vi "Read Discrete Inputs Request.vi"(8 "error in (no error)":errorcluster, 9 "number of inputs":u16, 10 "starting address":u16) -> (0 "error out":errorcluster, 1 "Modbus Data Unit out":T1={"function"=1, "Data"=[]} {"function" items=["Read Discrete Inputs"=2, "Read Coils"=1, "Write Single Coil"=5, "Write Multiple Coils"=15, "Read Input Register"=4, "Read Holding Registers"=3, "Write Single Register"=6, "Write Multiple Registers"=16, "Read/Write Multiple Registers"=23, "Mask Write Register"=22, "Read FIFO Queue"=24, "Read File Record"=20, "Write File Record"=21, "Read Exception Status"=7, "Diagnostic"=8, "Get Com Event Counter"=11, "Get Com Event Log"=12, "Report Slave ID"=17, "Read Device Identification"=43]; "Data" format="%.0x"})   [LabVIEW 2021, in "NI_modbus_upd.lvlib"]
doc: "This VI creates the modbus data unit for a read discrete inputs request."
uses:
  NI_modbus_upd.lvlib
  Ctl/MB Modbus Data Unit.ctl
  Modbus Data Unit (PDU)/Function.ctl
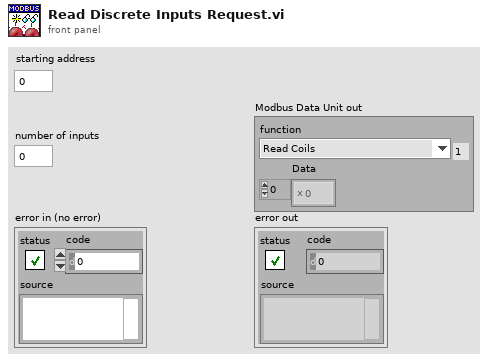
[diagram p1: front panel]
types:
  T1 = typedef "NI_modbus_upd.lvlib/MB Modbus Data Unit.ctl" = cluster{"function":T2, "Data":u8[]}
  T2 = typedef "NI_modbus_upd.lvlib/Function.ctl" = u8
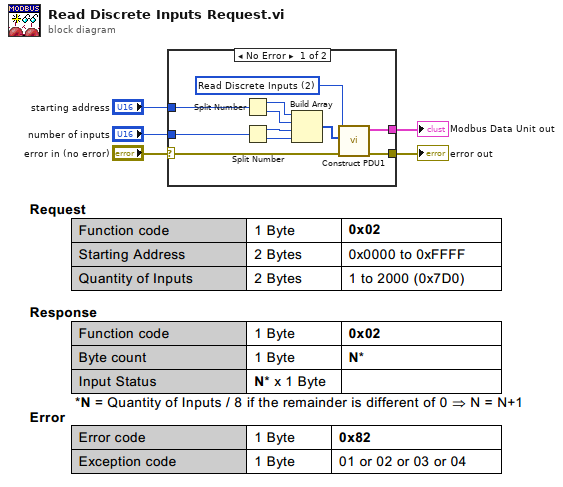
[diagram p0: block diagram]
diagram:
  n1 = case shown="No Error" "error in (no error)" {
    selector: "error in (no error)" -> [w6 w17]
    tunnel: [w16 w17] -> w5
    tunnel: "starting address" -> [w15 _]
    tunnel: "number of inputs" -> [w14 _]
    tunnel: [w13 _] -> w1
    frame No Error {
      w7 = T2 2 items=["Read Discrete Inputs"=2, "Read Coils"=1, "Write Single Coil"=5, "Write Multiple Coils"=15, "Read Input Register"=4, "Read Holding Registers"=3, "Write Single Register"=6, "Write Multiple Registers"=16, "Read/Write Multiple Registers"=23, "Mask Write Register"=22, "Read FIFO Queue"=24, "Read File Record"=20, "Write File Record"=21, "Read Exception Status"=7, "Diagnostic"=8, "Get Com Event Counter"=11, "Get Com Event Log"=12, "Report Slave ID"=17, "Read Device Identification"=43] ("Function")
      n2 = Split Number(x=w15) -> (hi(x)=w9:u8, lo(x)=w10:u8)
      n3 = Split Number(x=w14) -> (hi(x)=w11:u8, lo(x)=w12:u8)
      n4 = Build Array(w9, w10, w11, w12) -> (w8:u8[])
      n5 = call "Construct PDU1.vi"("error in (no error)"=w6, "data"=w8, "function"=w7) -> ("error out"=w16:errorcluster, "Modbus Data Unit out"=w13:T1)  [unwired: 7 in]
    }
    frame Error {
    }
  }
  "error out" <- w5
  "Modbus Data Unit out" <- w1
